vi "Save All.vi"(8 "error in (no error)":errorcluster, 10 "References":T1) -> (0 "error out":errorcluster)   [LabVIEW 2023, in "Message Maker.lvclass"]
doc: "Saves all items in the class\n\nAuthor: Derek Trepanier\nCopyright: MGI 2015"
uses:
  Message Maker.lvclass
  Message Maker.lvclass/Message Maker.ctl
  Scripting Refs.ctl
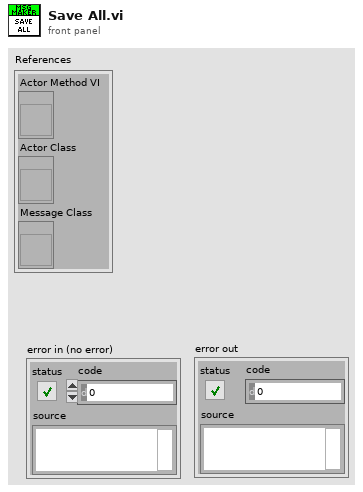
[diagram p1: front panel]
types:
  T1 = typedef "Message Maker.lvclass/Scripting Refs.ctl" = cluster{"Actor Method VI":refnum<vi>, "Actor Class":refnum<vi>, "Message Class":refnum<vi>}
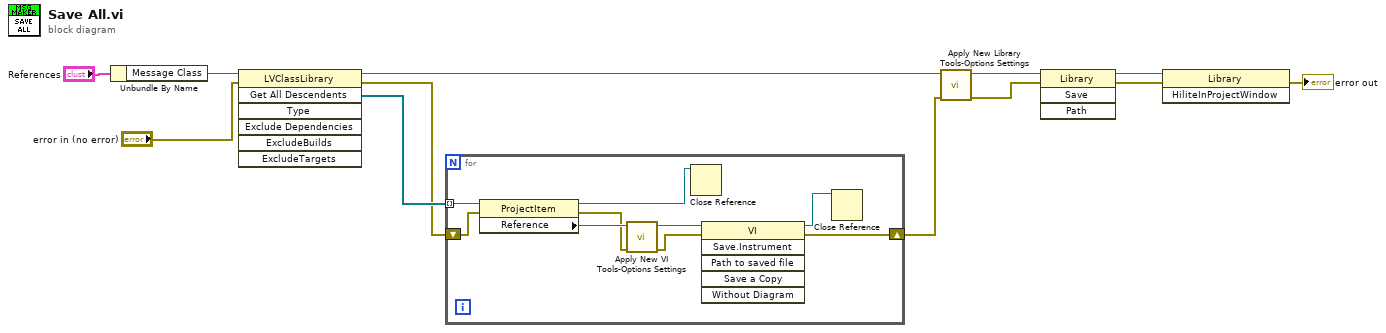
[diagram p0: block diagram]
diagram:
  n1 = Unbundle By Name("References") -> ("Message Class"=w11:refnum<vi>)
  n2 = invoke class="LVClassLibrary" method="Get All Descendents"(reference=w11, error in="error in (no error)") -> (reference out=w1:refnum<vi>, error out=w9:errorcluster, "All Descendents"=w10:refnum<vi>[])  [unwired: 5 in, 4 out]
  n3 = for {
    tunnel: w10 -> [w21] mode=indexing
    shift-right: [w20] -> w4
    shift-left: w9 -> [w19]
    n4 = property class="ProjectItem"(reference=w21, error in=w19) -> (reference out=w18:refnum<vi>, error out=w13:errorcluster, "Reference"=w16:refnum<vi>)
    n5 = call <vilib>:"Apply New VI Tools-Options Settings.vi"("error in (no error)"=w13, "VI Refnum"=w16) -> ("error out"=w14:errorcluster, "dup VI Refnum"=w15:refnum<vi>)  [unwired: 8 in]
    n6 = Close Reference(reference=w18) -> ()  [unwired: 1 in, 1 out]
    n7 = invoke class="VI" method="Save.Instrument"(reference=w15, error in=w14) -> (reference out=w17:refnum<vi>, error out=w20:errorcluster)  [unwired: 4 in, 4 out]
    n8 = Close Reference(reference=w17) -> ()  [unwired: 1 in, 1 out]
  }
  n9 = call <vilib>:"Apply New Library Tools-Options Settings.vi"("error in (no error)"=w4, "Library Refnum"=w1) -> ("error out"=w3:errorcluster, "dup Library Refnum"=w5:refnum<vi>)  [unwired: 8 in]
  n10 = invoke class="Library" method="Save"(reference=w5, error in=w3) -> (reference out=w8:refnum<vi>, error out=w7:errorcluster)  [unwired: 2 in, 2 out]
  n11 = invoke class="Library" method="HiliteInProjectWindow"(reference=w8, error in=w7) -> (error out=→"error out":errorcluster)  [unwired: 1 in, 2 out]
